vi "increment by factor rep2.vi"(4 "State":i16, 5 "Time":dbl format="%.2f", 6 "Sensor Values":dbl[](array[numeric]), 7 "Set Points":dbl[](array[numeric])) -> (0 "required data":T1={"Set Point names"=["reset state", "state to increment", "coefficient", "base", "max x", "reps"], "required number of setpoints"=6, "required number of sensors"=0, "Sensor names"=[]}, 3 "output value":dbl)   [LabVIEW 2019]
panel:
  # "Enter the correct information for this control code in the required data structure below. Then make the current value default by right clicking on the border of the data structure. Select \"data operations\" and then select \"make current value default\". These values will be displayed by process controller."
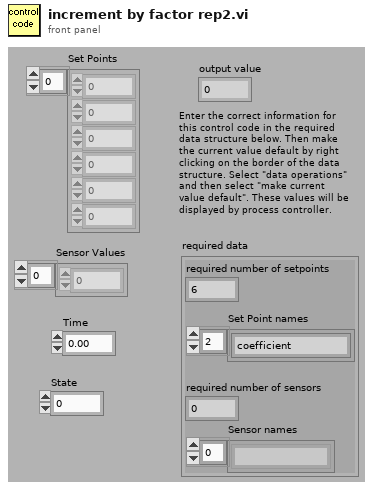
[diagram p1: front panel]
types:
  T1 = cluster{"Set Point names":string[], "required number of setpoints":u8, "required number of sensors":u8, "Sensor names":string[]}
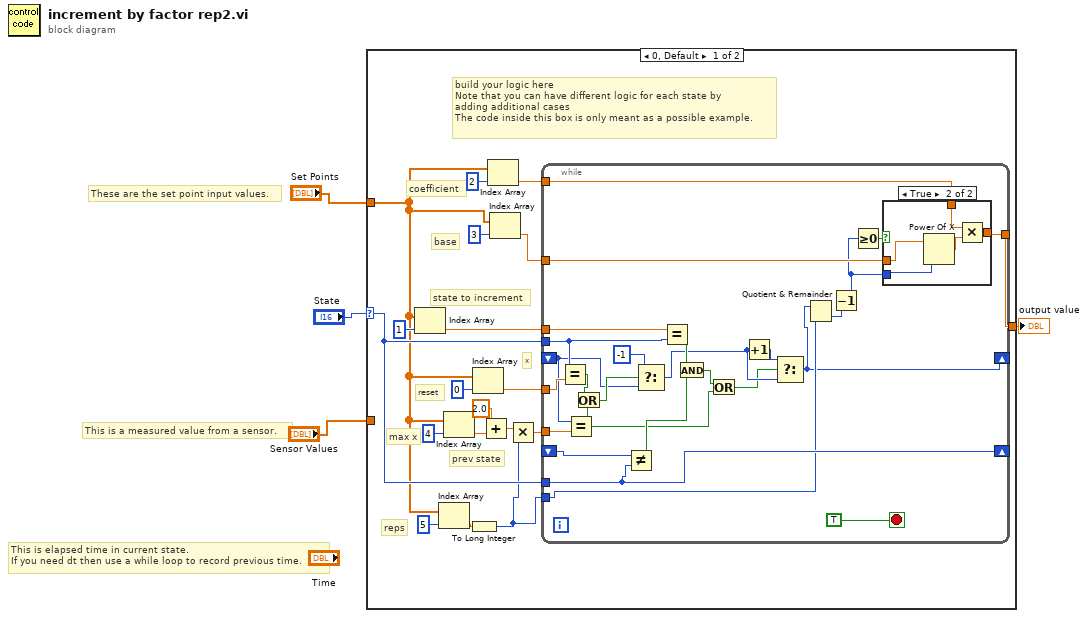
[diagram p0: block diagram]
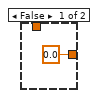
[diagram p2: hidden frame]
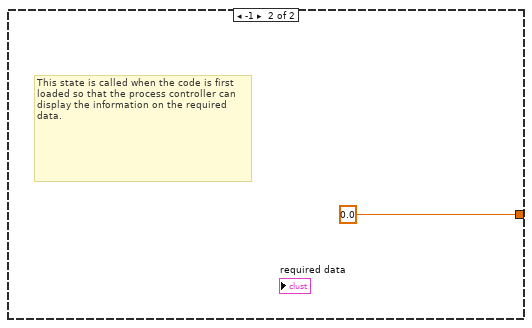
[diagram p3: hidden frame]
diagram:
  # "These are the set point input values."
  # "This is a measured value from a sensor."
  # "This is elapsed time in current state.\nIf you need dt then use a while loop to record previous time."
  n1 = case shown="0, Default" "State" {
    selector: "State" -> [w21 _]
    tunnel: [w18 0.0 ("fraction on")] -> w3
    tunnel: "Set Points" -> [w7 _]
    tunnel: "Sensor Values" -> [_ _]
    frame 0, Default {
      # "state to increment"
      # "coefficient"
      # "reps"
      # "max x"
      # "prev state"
      # "reset"
      # "base"
      # "x"
      # "build your logic here\nNote that you can have different logic for each state by\nadding additional cases\nThe code inside this box is only meant as a possible example."
      n2 = Index Array(array=w7, index=1) -> (element=w22:dbl)
      n3 = Index Array(array=w7, index=5) -> (element=w13:dbl)
      n4 = Index Array(array=w7, index=4) -> (element=w11:dbl)
      n5 = To Long Integer(number=w13) -> (32bit integer=w12:i32)
      n6 = Index Array(array=w7, index=0) -> (element=w16:dbl)
      n7 = Add(x=2.0, y=w11) -> (x+y=w10:dbl)
      n8 = Index Array(array=w7, index=2) -> (element=w6:dbl)
      n9 = Index Array(array=w7, index=3) -> (element=w19:dbl)
      n10 = Multiply(x=w10, y=w12) -> (x*y=w9:dbl)
      n11 = while {
        shift-right: [w48] -> _
        shift-left: _ -> [w40]
        tunnel: w21 -> [w48]
        tunnel: w22 -> [w49]
        tunnel: w21 -> [w43]
        shift-right: [w30] -> _
        shift-left: _ -> [w36]
        tunnel: w19 -> [w29]
        tunnel: [w28] -> w18
        tunnel: w16 -> [w42]
        tunnel: w9 -> [w39]
        tunnel: w12 -> [w31]
        tunnel: w6 -> [w27]
        stop <- TRUE stop-if-true
        n12 = Equal?(x=w43, y=w42) -> (x = y?=w38:bool)
        n13 = Equal?(x=w36, y=w39) -> (x = y?=w33:bool)
        n14 = Or(x=w38, y=w33) -> (x .or. y?=w37:bool)
        n15 = Not Equal?(x=w40, y=w48) -> (x != y?=w47:bool)
        n16 = Select(t=-1, s=w37, f=w36) -> (s? t:f=w41:i32)
        n17 = Equal?(x=w49, y=w43) -> (x = y?=w45:bool)
        n18 = And(x=w45, y=w47) -> (x .and. y?=w34:bool)
        n19 = Or(x=w34, y=w33) -> (x .or. y?=w32:bool)
        n20 = Increment(x=w41) -> (x+1=w44:i32)
        n21 = Select(t=w44, s=w32, f=w41) -> (s? t:f=w30:i32)
        n22 = Quotient & Remainder(x=w30, y=w31) -> (floor(x/y)=w25:i32)  [unwired: 1 out]
        n23 = Decrement(x=w25) -> (x-1=w24:i32)
        n24 = Greater Or Equal To 0?(x=w24) -> (x >= 0?=w26:bool)
        n25 = case shown="True" w26 {
          tunnel: w24 -> [_ w55]
          tunnel: w29 -> [_ w53]
          tunnel: [0.0 w52] -> w28
          tunnel: w27 -> [_ w51]
          frame False {
          }
          frame True {
            n26 = Power Of X(1:w53, 2:w55) -> (0:w54:dbl)
            n27 = Multiply(x=w51, y=w54) -> (x*y=w52:dbl)
          }
        }
      }
    }
    frame -1 {
      # "This state is called when the code is first loaded so that the process controller can display the information on the required data."
    }
  }
  "output value" <- w3
